vi "Scope.vi"(7 "JPG":refnum<vi>, 11 "Console Reference":refnum<vi>) -> ()   [LabVIEW 2020]
uses:
  <vilib>/Utility/file.llb/Write Delimited Spreadsheet (DBL).vi
panel:
  in  "start":bool
  in  "Save":bool
  in  "python":string
  in  "Send":bool
  in  "Clear":bool
  in  "Tab Control":enum32{"Scope", "XY Plot", "Gauges"}(tab)
  out "Graph":dbl[](graph)
  out "XY Plot":cluster{dbl[], dbl[]}[](graph)
  out "Gauge":dbl[](array[knob]) scale=-100.0..100.0
  out "Last Line":string
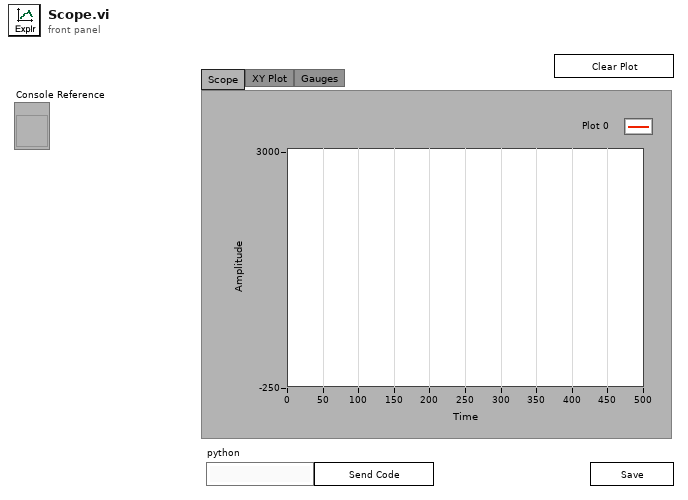
[diagram p1: front panel]
types:
  T1 = enum16{"Not data", "single values", "XY pairs", "Arrays"}
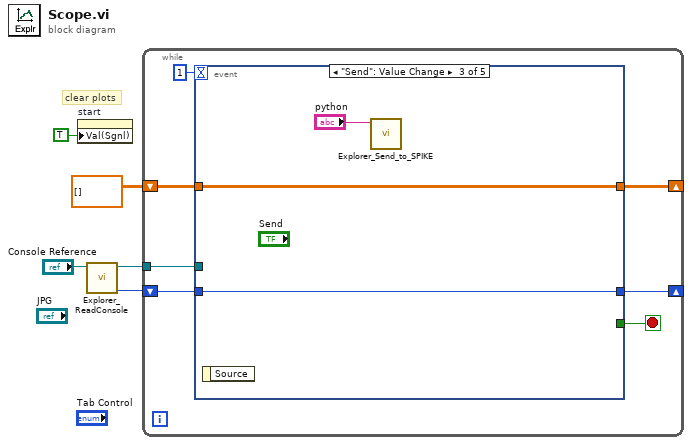
[diagram p0: block diagram]
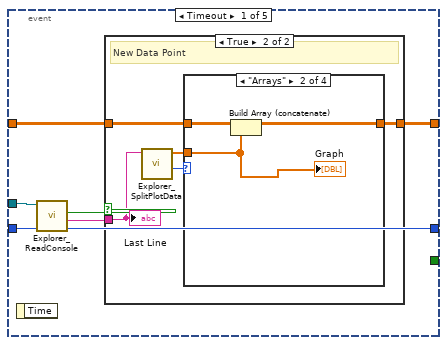
[diagram p2: hidden frame]
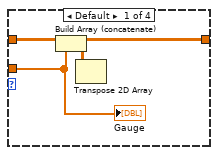
[diagram p4: hidden frame]
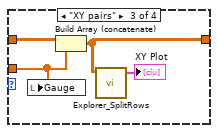
[diagram p5: hidden frame]
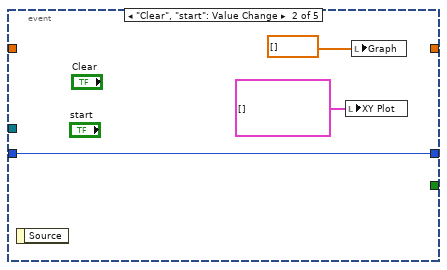
[diagram p7: hidden frame]
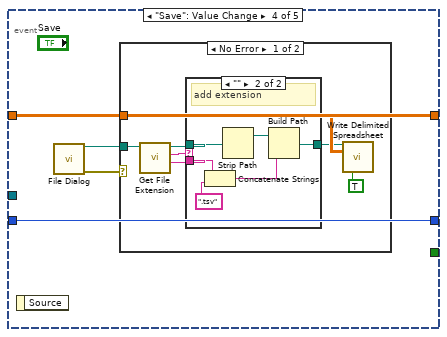
[diagram p8: hidden frame]
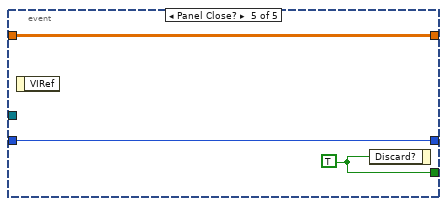
[diagram p11: hidden frame]
diagram:
  # "clear plots"
  n1 = property on="start" class="Bool (strict)"("Val(Sgnl)"=TRUE ("Value (Signaling)")) -> ()  [unwired: 2 in, 2 out]
  n2 = call "Explorer_ReadConsole.vi"("String in"="Console Reference") -> ("index out"=w4:i32, "String out"=w3:refnum<vi>)  [unwired: 6 in, 3 out]
  n3 = while {
    shift-right: [w10] -> _
    shift-left: w4 -> [w9]
    shift-right: [w7] -> _
    shift-left: dbl[][] [] -> [w8]
    tunnel: w3 -> [w6]
    stop <- w11 stop-if-true
    n4 = event shown="[2] \"Send\": Value Change" {
      selector: _ -> [_ _ _ _ _]
      dyn-events: _ -> [_ _ _ _ _]
      timeout: 1 -> [_ _ _ _ _]
      tunnel: [_ _ _ _ w63] -> w11
      tunnel: [w16 w39 w41 w46 w62] -> w10
      tunnel: w9 -> [w17 w39 w41 w46 w62]
      tunnel: w8 -> [w19 _ w42 w45 w61]
      tunnel: [w18 _ w42 w45 w61] -> w7
      tunnel: w6 -> [w13 _ _ _ _]
      event Timeout {
        n5 = event-data() -> ()  [unwired: 1 in, 1 out]
        n6 = call "Explorer_ReadConsole.vi"("index in"=w17, "String in"=w13) -> ("index out"=w16:i32, "New Line"=w15:string, "New point?"=w14:bool)  [unwired: 5 in, 2 out]
        n7 = case shown="True" w14 {
          tunnel: w15 -> [_ w25]
          tunnel: w19 -> [w20 w24]
          tunnel: [w20 w23] -> w18
          frame False {
            # "nothing new"
          }
          frame True {
            # "New Data Point"
            n8 = call "Explorer_SplitPlotData.vi"("Value"=w25) -> ("Data type"=w22:T1, "Array"=w21:dbl[])  [unwired: 9 in]
            n9 = case shown="\"Arrays\"" w22 {
              tunnel: w24 -> [w28 w31 w35 w36]
              tunnel: [w27 w30 w34 w36] -> w23
              tunnel: w21 -> [w26 w29 w32 _]
              frame Default {
                n10 = Build Array (concatenate)(w28, w26) -> (w27:dbl[][])
                n11 = Transpose 2D Array(2D array=w27) -> ()  [unwired: 1 out]
                "Gauge" <- w26
              }
              frame "Arrays" {
                n12 = Build Array (concatenate)(w31, w29) -> (w30:dbl[][])
                "Graph" <- w29
              }
              frame "XY pairs" {
                n13 = local write "Gauge"(w32) -> ()
                n14 = Build Array (concatenate)(w35, w32) -> (w34:dbl[][])
                n15 = call "Explorer_SplitRows.vi"("Array in"=w34) -> ("XY Plot"=→"XY Plot":cluster{dbl[], dbl[]}[])  [unwired: 10 in]
              }
              frame "Not data" {
              }
            }
            "Last Line" <- w25
          }
        }
      }
      event "Clear", "start": Value Change {
        n16 = event-data() -> ()  [unwired: 1 in, 1 out]
        n17 = local write "XY Plot"(cluster{dbl[], dbl[]}[] [] ("XY Plot")) -> ()
        n18 = local write "Graph"(dbl[] []) -> ()
      }
      event "Send": Value Change {
        n19 = event-data() -> ()  [unwired: 1 in, 1 out]
        n20 = call "Explorer_Send_to_SPIKE.vi"("python"="python") -> ()  [unwired: 10 in, 1 out]
      }
      event "Save": Value Change {
        n21 = event-data() -> ()  [unwired: 1 in, 1 out]
        n22 = call "File Dialog"() -> ("selected path"=w44:path, "error out"=w43:errorcluster)  [unwired: 12 in, 2 out]
        n23 = case shown="No Error" w43 {
          tunnel: w45 -> [w53 _]
          tunnel: w44 -> [w51 _]
          frame No Error {
            n24 = call <vilib>:"Get File Extension.vi"("file"=w51) -> ("filename without extension"=w47:string, "lowercase file extension"=w50:string, "dup file"=w48:path)  [unwired: 6 in, 2 out]
            n25 = case shown="\"\"" w50 {
              tunnel: [w54 w56] -> w49
              tunnel: w48 -> [w54 w58]
              tunnel: w47 -> [_ w60]
              frame Default {
              }
              frame "" {
                # "add extension"
                n26 = Concatenate Strings(w60, ".tsv" ("pattern (all files)")) -> (w55:string)
                n27 = Strip Path(path=w58) -> (stripped path=w57:path)  [unwired: 1 out]
                n28 = Build Path(base path=w57, name or relative path=w55) -> (appended path=w56:path)
              }
            }
            n29 = call-poly <vilib>:"Write Delimited Spreadsheet.vi"("file path (dialog if empty)"=w49, "2D data"=w53, "transpose? (no:F)"=TRUE) -> ()  [unwired: 11 in, 2 out]
          }
          frame Error {
          }
        }
      }
      event Panel Close? {
        w63 = TRUE ("Discard?")
        n30 = event-data() -> ()  [unwired: 1 in, 1 out]
        n31 = event-data("Discard?"=w63) -> ()  [unwired: 1 in, 1 out]
      }
    }
  }
